vi "Test Set PSU X.vi"(8 "error in (no error)":errorcluster, 11 "Instrument.OxfordVRM in":refnum<class "Instrument.OxfordVRM.lvclass">) -> (0 "error out":errorcluster, 3 "Instrument.OxfordVRM out":refnum<class "Instrument.OxfordVRM.lvclass">)   [LabVIEW 2016, in "Instrument.OxfordVRM.lvclass"]
uses:
  Instrument.OxfordVRM.lvclass
  <vilib>/addons/_JKI Toolkits/Caraya/classes/Assert/Assert Not Error.vi
  <vilib>/addons/_JKI Toolkits/Caraya/classes/Assert/Assert Equal Value and Type_Variant.vi
  <vilib>/addons/_JKI Toolkits/Caraya/classes/Test/Test.lvclass
  <vilib>/addons/_JKI Toolkits/Caraya/classes/Assert/Assert.lvclass
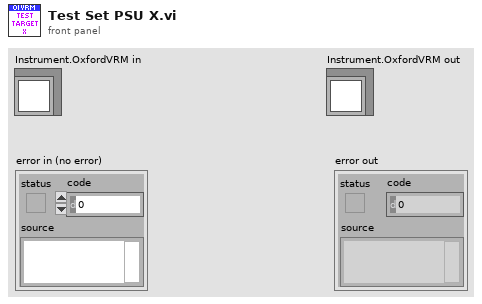
[diagram p1: front panel]
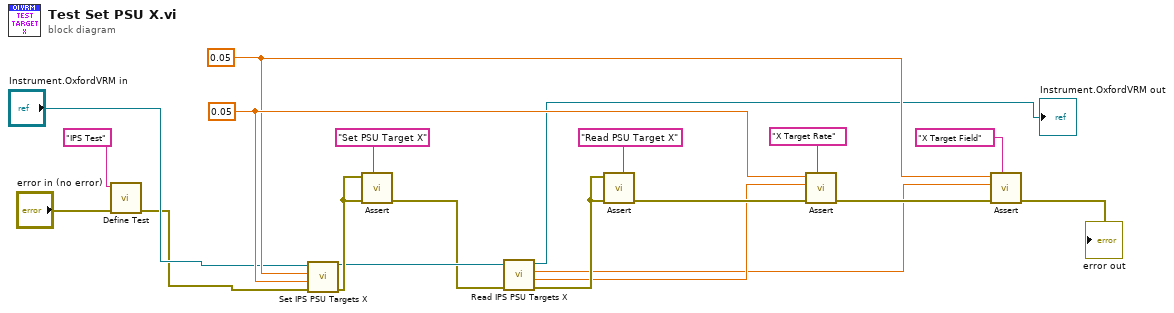
[diagram p0: block diagram]
diagram:
  w9 = 0.05 ("Target Field Rate (T/min)")
  w7 = 0.05 ("Target Field (T)")
  n1 = call <vilib>:"Define Test.vi"("error in (no error)"="error in (no error)", "Label (VI Title)"="IPS Test") -> ("error out"=w1:errorcluster)  [unwired: 9 in]
  n2 = call "Set IPS PSU Targets X.vi"("error in (no error)"=w1, "Target Field Rate (T/min)"=w9, "Target Field (T)"=w7, "Instrument.OxfordVRM in"="Instrument.OxfordVRM in") -> ("error out"=w19:errorcluster, "Instrument.OxfordVRM out"=w17:refnum<class "Instrument.OxfordVRM.lvclass">)  [unwired: 5 in, 1 out]
  n3 = call-poly <vilib>:"Assert.vi"("Label"="Set PSU Target X", "error in (no error)"=w19, "Not Error?"=w19) -> ("error out"=w16:errorcluster)  [unwired: 8 in]
  n4 = call "Read IPS PSU Targets X.vi"("error in (no error)"=w16, "Instrument.OxfordVRM in"=w17) -> ("error out"=w15:errorcluster, "Target Field Rate (T/min)"=w8:dbl, "Target Field (T)"=w6:dbl, "Instrument.OxfordVRM out"=→"Instrument.OxfordVRM out":refnum<class "Instrument.OxfordVRM.lvclass">)  [unwired: 6 in]
  n5 = call-poly <vilib>:"Assert.vi"("Label"="Read PSU Target X", "error in (no error)"=w15, "Not Error?"=w15) -> ("error out"=w12:errorcluster)  [unwired: 8 in]
  n6 = call-poly <vilib>:"Assert.vi"("Label"="X Target Rate", "error in (no error)"=w12, "Y"=w8, "X"=w9) -> ("error out"=w11:errorcluster)  [unwired: 7 in]
  n7 = call-poly <vilib>:"Assert.vi"("Label"="X Target Field", "error in (no error)"=w11, "Y"=w6, "X"=w7) -> ("error out"=→"error out":errorcluster)  [unwired: 7 in]
